vi "Configure Arbitrary Waveform Phase.vi"(7 "Units (0: Degree)":i32(ring) items=["Degree", "Radian", "Second", "Sample"], 8 "error in (no error)":errorcluster, 9 "Phase Offset (0 Degree)":dbl, 10 "Channel (1: 1)":i32(ring)=1 items=["1"=1, "2"=2], 11 "VISA resource name":refnum<visa-resource-name>) -> (0 "error out":errorcluster, 3 "VISA resource name out":refnum<visa-resource-name>)   [LabVIEW 2019, in "Agilent 3352X Series.lvlib"]
doc: "Sets the offset for the currently selected arbitrary waveform in either degrees, radians, seconds or samples.\n\n<b>Note</b>: \n(1) This VI is only applicable for 33611A, 33612A, 33621A and 33622A models and arbitrary waveforms of at least 64 samples.\n(2) This VI affects the phase of the currently selected arbitrary waveform only.\n(3) This VI affects the phase of the arbitrary in normal continuous mode, modulation mode, and sweep mode but not burst mode.\n(4) When an arbitrary waveform is loaded into memory, its initial phase is zero; it does not inherit the phase of the currently selected arbitrary waveform. Each arbitrary waveform retains its own phase setting while in memory.\n(5) The phase of the arbitrary waveform is defined with respect to all the points in the arbitrary waveform record."
uses:
  Agilent 3352X Series.lvlib
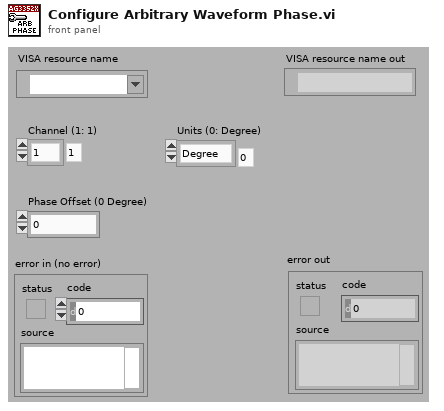
[diagram p1: front panel]
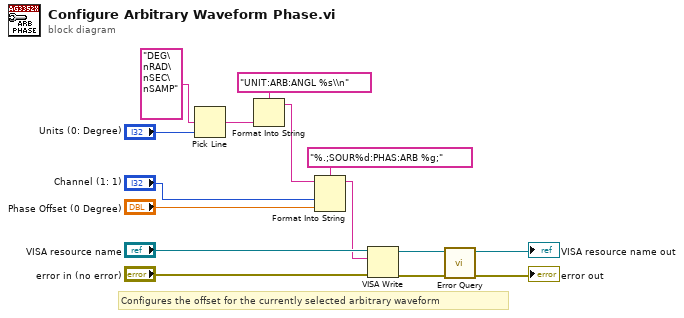
[diagram p0: block diagram]
diagram:
  # "Configures the offset for the currently selected arbitrary waveform"
  n1 = Pick Line(multi-line string="DEG\nRAD\nSEC\nSAMP", line index="Units (0: Degree)") -> (output string=w3:string)  [unwired: 1 out]
  n2 = Format Into String(format string="UNIT:ARB:ANGL %s\\n", w3) -> (resulting string=w1:string)  [unwired: 2 in, 1 out]
  n3 = Format Into String(format string="%.;SOUR%d:PHAS:ARB %g;", initial string=w1, "Channel (1: 1)", "Phase Offset (0 Degree)") -> (resulting string=w8:string)  [unwired: 1 in, 1 out]
  n4 = VISA Write(VISA resource name="VISA resource name", write buffer=w8, error in (no error)="error in (no error)") -> (VISA resource name out=w12:refnum<visa-resource-name>, error out=w11:errorcluster)  [unwired: 1 out]
  n5 = call "Error Query.vi"("error in (no error)"=w11, "VISA resource name"=w12) -> ("error out"=→"error out":errorcluster, "VISA resource name out"=→"VISA resource name out":refnum<visa-resource-name>)  [unwired: 8 out]
